vi "Auto indexing.vi"() -> ()   [LabVIEW 2018]
panel:
  out "Array 6":dbl[][](array[numeric])
  out "Array 4":dbl[](array[numeric])
  out "Array 3":dbl[](array[numeric])
  out "Array 2":dbl[](array[numeric])
  out "Numeric":dbl
  out "Array":dbl[](array[numeric])
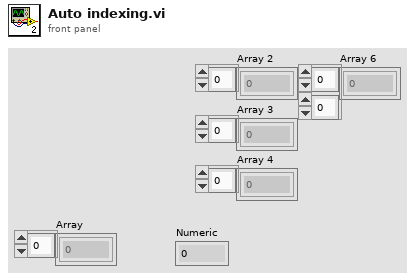
[diagram p1: front panel]
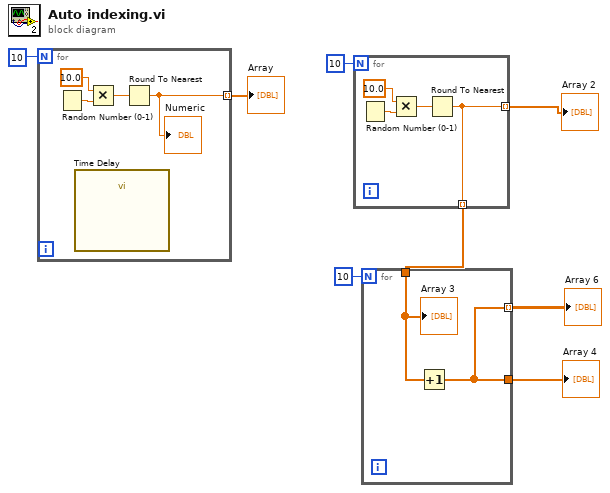
[diagram p0: block diagram]
diagram:
  n1 = for {
    N: 10 -> [_]
    tunnel: [w9] -> w7 mode=indexing
    n2 = Random Number (0-1)() -> (number: 0 to 1=w12:dbl)
    n3 = call "Time Delay"() -> ()  [unwired: 11 in, 1 out]
    n4 = Multiply(x=10.0, y=w12) -> (x*y=w10:dbl)
    n5 = Round To Nearest(number=w10) -> (nearest integer value=w9:dbl)
    "Numeric" <- w9
  }
  "Array" <- w7
  n6 = for {
    N: 10 -> [_]
    tunnel: [w13] -> w5 mode=indexing
    tunnel: [w13] -> w3 mode=indexing
    n7 = Random Number (0-1)() -> (number: 0 to 1=w16:dbl)
    n8 = Multiply(x=10.0, y=w16) -> (x*y=w15:dbl)
    n9 = Round To Nearest(number=w15) -> (nearest integer value=w13:dbl)
  }
  "Array 2" <- w5
  n10 = for {
    N: 10 -> [_]
    tunnel: w3 -> [w18]
    tunnel: [w17] -> w2
    tunnel: [w17] -> w1 mode=indexing
    n11 = Increment(x=w18) -> (x+1=w17:dbl[])
    "Array 3" <- w18
  }
  "Array 4" <- w2
  "Array 6" <- w1
